vi "FromIPrinter.vi"(10 "OT3IPrinter":refnum<class "OT3IPrinter.lvclass">) -> (3 "OfficeTron3000":refnum<class "OfficeTron3000.lvclass">)   [LabVIEW 2018, in "OfficeTron3000.lvlib" / "OfficeTron3000.lvclass"]
uses:
  OfficeTron3000.lvclass
  OT3IPrinter/OT3IPrinter.lvclass
  OT3IPrinter/OT3IPrinter.lvclass/OT3IPrinter.ctl
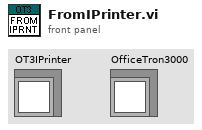
[diagram p1: front panel]
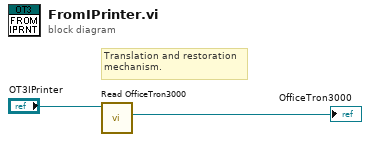
[diagram p0: block diagram]
diagram:
  # "Translation and restoration\nmechanism."
  n1 = call "Read OfficeTron3000.vi"("OT3IPrinter In"="OT3IPrinter") -> ("OfficeTron3000"=→"OfficeTron3000":refnum<class "OfficeTron3000.lvclass">)  [unwired: 9 in, 1 out]
